vi "Build Message.vi"(8 "error in (no error)":errorcluster, 10 "Data to Send":u8[](array[numeric]) format="%.0x", 11 "EF20 in":refnum<class "EF20.lvclass">) -> (0 "error out":errorcluster, 3 "EF20 out":refnum<class "EF20.lvclass">)   [LabVIEW 2018, in "EF20.lvlib" / "EF20.lvclass"]
uses:
  EF20.lvclass
  EF20.lvclass/EF20.ctl
panel:
  out "string":string
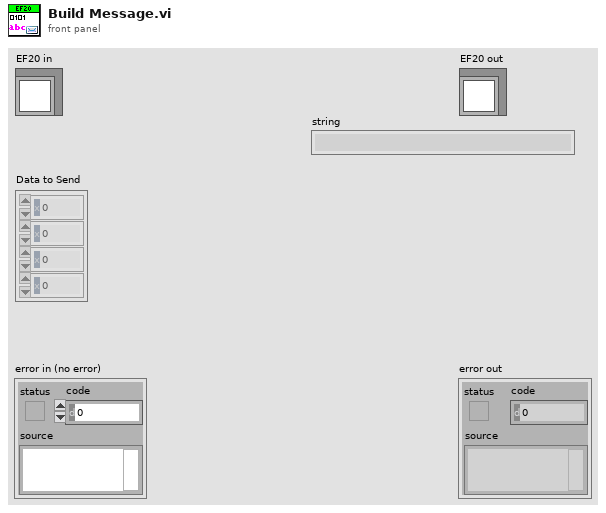
[diagram p1: front panel]
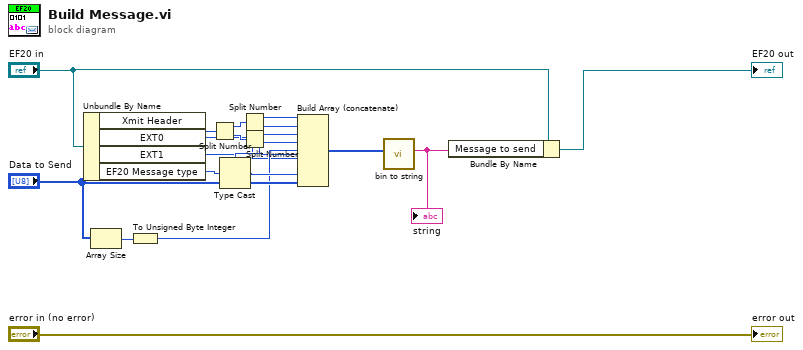
[diagram p0: block diagram]
diagram:
  n1 = Unbundle By Name("EF20 in") -> ("Xmit Header"=w17:u32, "EXT0"=w2:u8, "EXT1"=w1:u8, "EF20 Message type"=w3:u8)
  n2 = Array Size(array="Data to Send") -> (size(s)=w9:i32)
  n3 = To Unsigned Byte Integer(number=w9) -> (unsigned 8bit integer=w4:u8)
  n4 = Split Number(x=w17) -> (hi(x)=w18:u16, lo(x)=w7:u16)
  n5 = Split Number(x=w18) -> (hi(x)=w16:u8, lo(x)=w15:u8)
  n6 = Split Number(x=w7) -> (hi(x)=w14:u8, lo(x)=w6:u8)
  n7 = Type Cast(type=w6, x=w3) -> (*(type *) &x=w8:u8)
  n8 = Build Array (concatenate)(w16, w15, w14, w6, w4, w2, w1, w8, "Data to Send") -> (w12:u8[])
  n9 = call "bin to string.vi"("Data in"=w12) -> ("string"=w10:string)  [unwired: 10 in]
  "string" <- w10
  n10 = Bundle By Name(cluster="EF20 in", "Message to send"=w10) -> (→"EF20 out":refnum<class "EF20.lvclass">)
  "error out" <- "error in (no error)"
